vi "Dispose.vi"(8 "error in (no error)":errorcluster, 11 "DoorNeedingSpell":refnum<class "DoorNeedingSpell.lvclass">) -> (0 "error out":errorcluster)   [LabVIEW 2020, in "DoorNeedingSpell.lvclass"]
uses:
  DoorNeedingSpell.lvclass
  DoorNeedingSpell.lvclass/DoorNeedingSpell.ctl
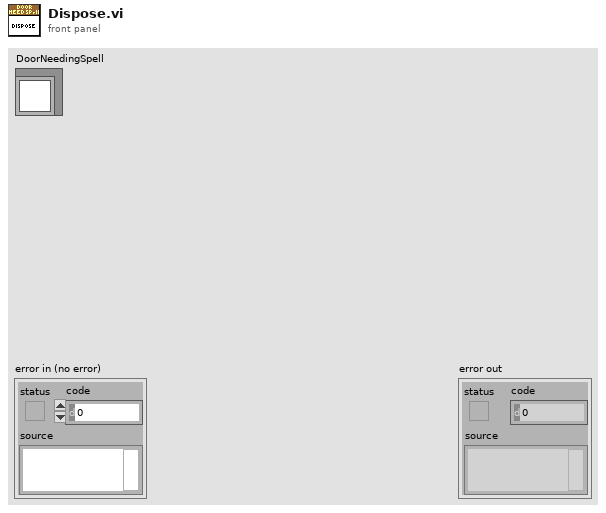
[diagram p1: front panel]
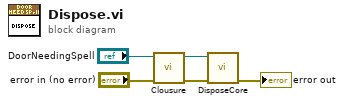
[diagram p0: block diagram]
diagram:
  n1 = call-dynamic "Clousure.vi"("error in (no error)"="error in (no error)", "DoorNeedingSpell"="DoorNeedingSpell") -> ("error out"=w1:errorcluster, "DoorNeedingSpell"=w2:refnum<class "DoorNeedingSpell.lvclass">)  [unwired: 8 in]
  n2 = call-dynamic "DisposeCore.vi"("error in (no error)"=w1, "DoorNeedingSpell"=w2) -> ("error out"=→"error out":errorcluster)  [unwired: 8 in, 1 out]
